vi "ESP301_Go2Pos.vi"(0 "VISA resource name":refnum<visa-resource-name>, 1 "Set value":dbl, 2 "Axis (1)":i32=1 min=1 max=3, 3 "Error In":errorcluster, 4 "DigNum Refnum":refnum<vi>) -> (5 "VISA resource name 2":refnum<visa-resource-name>, 6 "Error In 2":errorcluster)   [LabVIEW 2019]
uses:
  Newport ESP301/Newport ESP301.lvlib
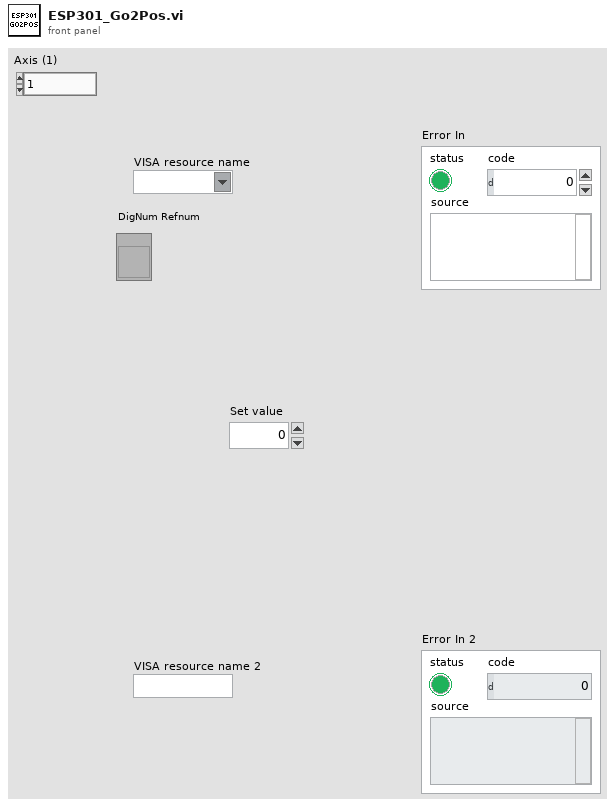
[diagram p1: front panel]
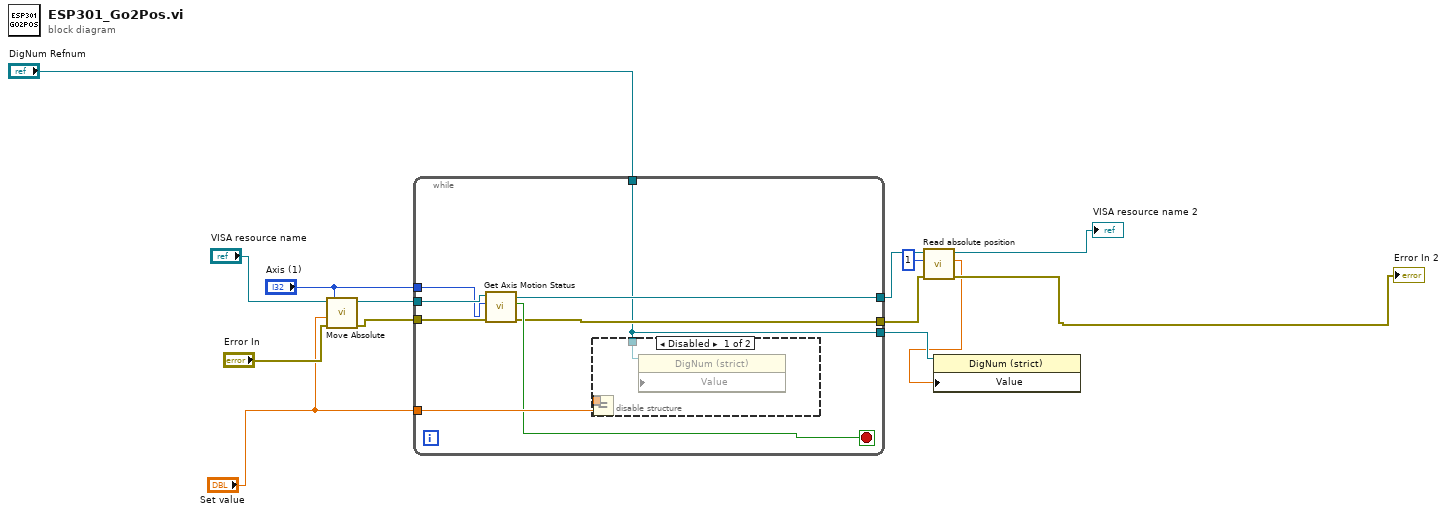
[diagram p0: block diagram]
diagram:
  n1 = call "Move Absolute.vi"("error in (no error)"="Error In", "Position (0 units)"="Set value", "Axis (1)"="Axis (1)", "VISA resource name"="VISA resource name") -> ("error out"=w12:errorcluster, "VISA resource name out"=w9:refnum<visa-resource-name>)  [unwired: 2 in]
  n2 = while {
    tunnel: w9 -> [w22]
    tunnel: w12 -> [w21]
    tunnel: "Axis (1)" -> [w20]
    tunnel: [w16] -> w7
    tunnel: [w17] -> w5
    tunnel: "Set value" -> [w19]
    tunnel: "DigNum Refnum" -> [w15]
    tunnel: [w15] -> w2
    stop <- w18 stop-if-true
    n3 = call "Get Axis Motion Status.vi"("error in (no error)"=w21, "Axis (1)"=w20, "VISA resource name"=w22) -> ("error out"=w17:errorcluster, "Motion Done"=w18:bool, "VISA resource name out"=w16:refnum<visa-resource-name>)  [unwired: 2 in]
    n4 = disable-structure shown="Disabled" {
      disable-tunnel: w19 -> [w25 _]
      disable-tunnel: w15 -> [w24 _]
      disable-tunnel: _ -> [w23 _]
      frame Disabled {
        n5 = Equal?(x=w23, y=w25) -> ()  [unwired: 1 out]
        n6 = property class="DigNum (strict)" props=["Value"](reference=w24) -> ()  [unwired: 2 in, 2 out]
      }
      frame Enabled {
      }
    }
  }
  n7 = call "Read absolute position.vi"("error in (no error)"=w5, "Axis (1)"=1, "VISA resource name"=w7) -> ("error out"=→"Error In 2":errorcluster, "Position (units)"=w1:dbl, "VISA resource name out"=→"VISA resource name 2":refnum<visa-resource-name>)  [unwired: 2 in]
  n8 = property class="DigNum (strict)"(reference=w2, "Value"=w1) -> ()  [unwired: 1 in, 2 out]
